vi "LIA_FPGA.vi"() -> ()   [LabVIEW 2010]
uses:
  <vilib>/rvi/LocalResourceManager/LocalResourceManager.xnode
  <vilib>/rvi/DataTransferAndStorage/Container/Common/niFpgaContainerState.ctl
  <vilib>/rvi/DataTransferAndStorage/Container/Common/niFpgaDataTypeControl.ctl
  <vilib>/rvi/DataTransferAndStorage/Container/Common/niFpgaContainerImplementationControl.ctl
  <vilib>/rvi/DataTransferAndStorage/Container/Common/niFpgaContainerArbitrationOptionsControl.ctl
  <vilib>/rvi/DataTransferAndStorage/Container/Common/niFpgaTransferTypeControl.ctl
  <vilib>/rvi/DataTransferAndStorage/Container/Common/niFpgaContainerInitializationParameters.ctl
  <vilib>/rvi/Memory/Memory_Types/niFpgaMemoryInterfaceConfiguration.ctl
  <vilib>/rvi/FIFO/Fifo_Types/niFpgaFifoControlLogicControl.ctl
  <vilib>/rvi/DataTransferAndStorage/Container/Common/niFpgaContainerMetaDataKey.ctl
  <vilib>/Platform/TimedLoop/XDataNode/XDataNode.xnode
  <vilib>/Platform/TimedLoop/XDataNode/timing_clust.ctl
  <vilib>/Platform/TimedLoop/XDataNode/nitl_modes.ctl
  <vilib>/Platform/TimedLoop/XDataNode/wakeup.ctl
  <vilib>/rvi/DataTransferAndStorage/Container/XNode/niFpgaContainer.xnode
  <vilib>/rvi/FXPMathLib/FxpInterpret/XNode/nifxpmath_Interpret.xnode
  <vilib>/eio/EIONode/EIONode.xnode
  <vilib>/rvi/eio/nirviEIOImplementation/nirviEIOImplementation.xnode
  <vilib>/rvi/eio/common/nirviEmuClasses.ctl
  <vilib>/rvi/DataTransferAndStorage/Container/Common/niFpgaContainerGetUniqueNameForEmu.vi
  <vilib>/rvi/DataTransferAndStorage/Container/Common/niFpgaContainerSetEmuInfo.vi
  <vilib>/rvi/eio/common/nirviEmuReportErrorAndStop.vi
  <vilib>/rvi/FIFO/Fifo_Resource/nirvififoEmulationSetSize.vi
  <vilib>/rvi/eio/common/nirviEmuTemplateMethod_noerrors.vi
  <vilib>/Platform/TimedLoop/XDataNode/XDNodeRunTimeDep.lvlib
panel:
  in  "Period":u16=1000
  out "ticks":u16
  out "ref":i16 format="%.0x"
  out "sig":i16 format="%.0x"
  out "channelQ":i64
  out "channelI":i64
  out "f":fxp<+/-,32,0> format="%.32g"
  in  "start":bool
  in  "dec2":i16=1
  in  "K":fxp<+,16,0>=0.001007080078125
  in  "nominal freq":fxp<+,16,0>=0.010009765625
  in  "dec1":i16=1
  in  "stages":i8=1
  in  "stop":bool
  in  "decimation":i16=1024
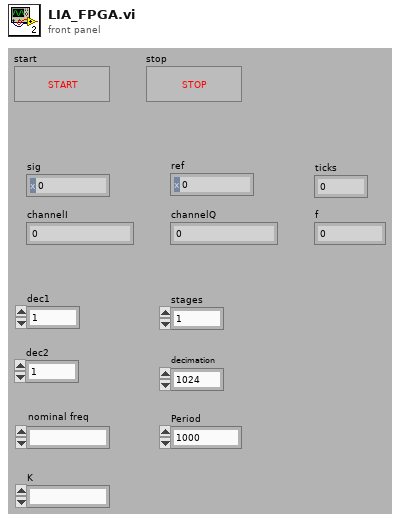
[diagram p1: front panel]
types:
  T1 = typedef "nirviEmuClasses.ctl" = enum16{"IO Read", "IO Write", "Method", "Property Read", "Property Write"}
  T2 = typedef "XDNodeRunTimeDep.lvlib/timing_clust.ctl" = cluster{"Expected End [f-1]":u64, "Actual End [f-1]":u64, "Finished Late? [f-1]":bool, "Expected End [i-1]":u64, "Actual End [i-1]":u64, "Finished Late? [i-1]":bool, "Expected Start [i]":u64, "Actual Start [i]":u64, "Expected Start [f]":u64, "Actual Start [f]":u64, "Source Name":string, "Structure Name":string, "Period":i64, "Deadline":i64, "Offset":i64, "Start":i64, "Priority":i32, "Timeout":i32, "Mode":T3, "Wakeup Reason":T4, "Error":errorcluster, "Source Type":string, "Secondary Source Type":string, "Global End Time":u64, "Global Start Time":u64, "Frame Duration":u64, "Iteration Duration":u64, "Assigned CPU":i32, "I/O Scan Engine Mode":u32}
  T3 = typedef "XDNodeRunTimeDep.lvlib/nitl_modes.ctl" = enum32{"No Change", "Process missed periods, maintain original phase", "Discard missed periods, maintain original phase", "Process missed periods, ignore original phase", "Discard missed periods, ignore original phase"}
  T4 = typedef "XDNodeRunTimeDep.lvlib/wakeup.ctl" = enum32{"Normal", "Aborted", "Asynchronous wakeup", "Timing source error", "Timed loop error", "Timeout"}
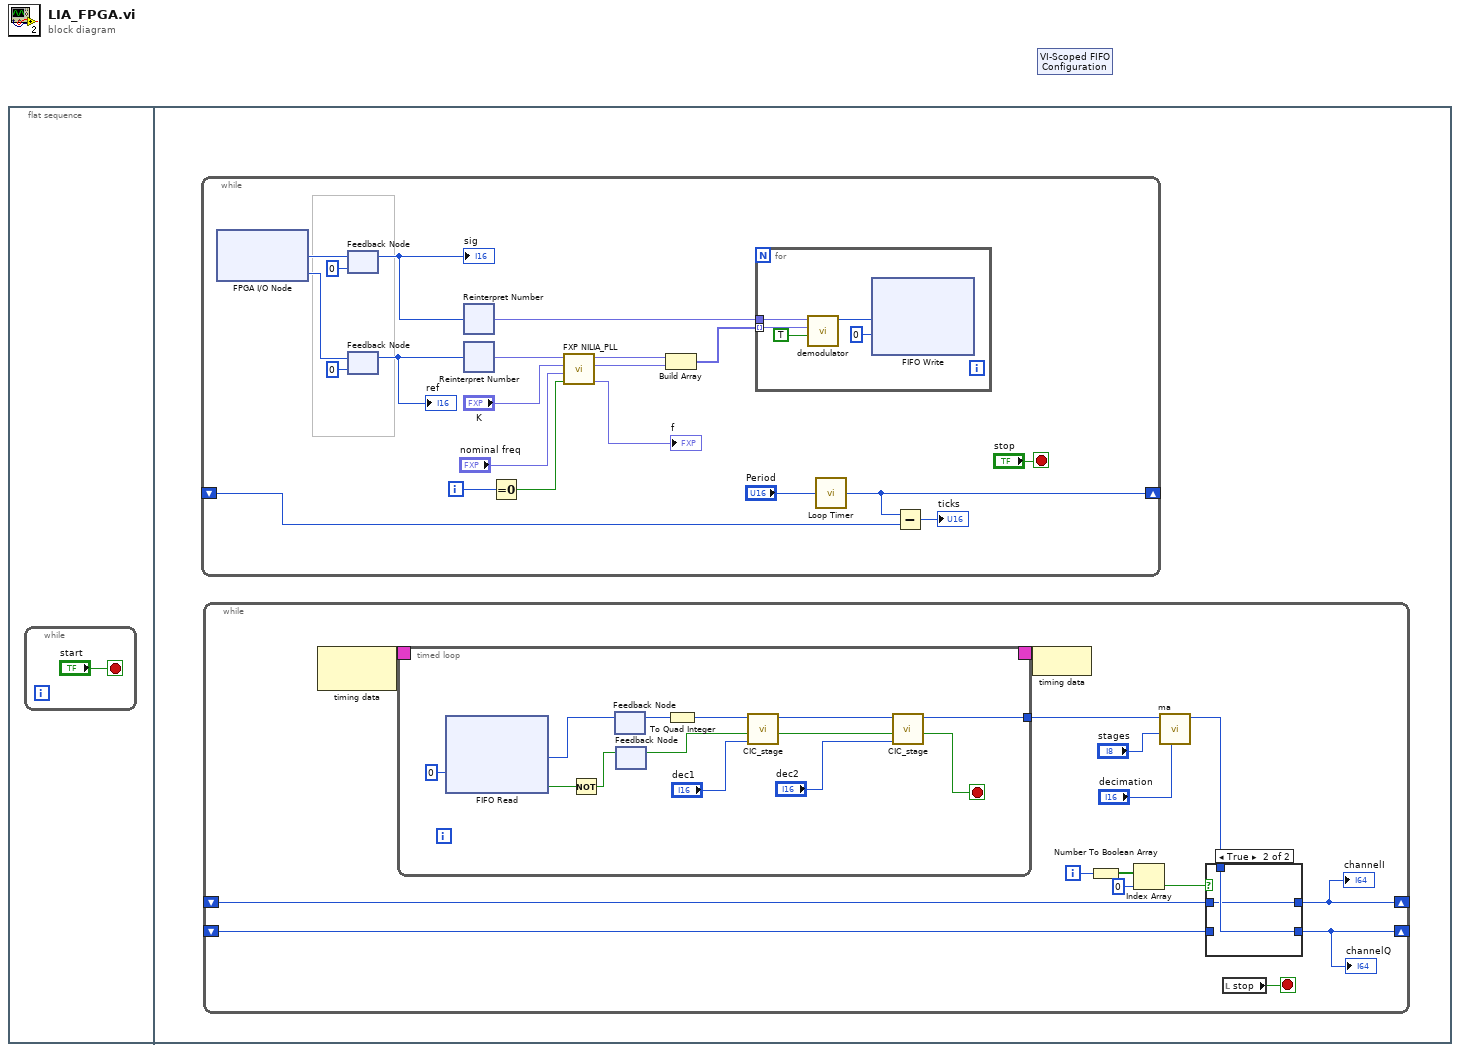
[diagram p0: block diagram]
diagram:
  n1 = flat-sequence {
    frame #0 {
      n2 = while {
        stop <- "start" stop-if-true
      }
    }
    frame #1 {
      n3 = while {
        shift-right: [w15] -> _
        shift-left: _ -> [w14]
        i -> [w22]
        stop <- "stop" stop-if-true
        n4 = xnode "FPGA I/O Node"() -> ("ModA/AI0"=w7:i16, "ModA/AI1"=w4:i16)  [unwired: 2 in, 2 out]
        n5 = feedback #1(i16 0 ("y")) -> (w6:i16)
        "sig" <- w6
        n6 = feedback-in #1(w7) -> ()
        n7 = feedback #2(i16 0 ("z [I32.1]")) -> (w5:i16)
        "ref" <- w5
        n8 = feedback-in #2(w4) -> ()
        n9 = xnode "Reinterpret Number"("x"=w6) -> ("y"=w10:fxp<+/-,16,1>)
        n10 = xnode "Reinterpret Number"("x"=w5) -> ("y"=w12:fxp<+/-,16,1>)
        n11 = Equal To 0?(x=w22) -> (x = 0?=w20:bool)
        n12 = call "FXP NILIA_PLL.vi"("reset?"=w20, "norminal freq [U16.0]"="nominal freq", "alpha [U16.0]"="K", "x[I16.1]"=w12) -> ("f"=→"f":fxp<+/-,32,0>, "sin(z)"=w2:fxp<+/-,16,2>, "cos(z)"=w3:fxp<+/-,16,2>)  [unwired: 1 in, 4 out]
        n13 = Build Array(w3, w2) -> (w11:fxp<+/-,16,2>[])
        n14 = for {
          tunnel: w10 -> [w25]
          tunnel: w11 -> [w23] mode=indexing
          n15 = call "demodulator.vi"("New Data"=TRUE, "ref"=w23, "signal"=w25) -> ("x*y"=w26:i32)  [unwired: 8 out]
          n16 = xnode ("FIFO Write")("Element"=w26, "Timeout"=0) -> ()  [unwired: 1 in, 2 out]
        }
        n17 = call "Loop Timer"("Count(Ticks)"="Period") -> ("Tick Count(Ticks)"=w15:u16)
        n18 = Subtract(x=w15, y=w14) -> (x-y=→"ticks":u16)
      }
      n19 = while {
        shift-right: [w122] -> _
        shift-left: _ -> [w124]
        shift-right: [w121] -> _
        shift-left: _ -> [w123]
        i -> [w129]
        stop <- w131 stop-if-true
        n20 = node-c288() -> (w135:T2)  [unwired: 1 out]
        n21 = timed-loop {
          timing: w135 -> [_]
          timing-out: [_] -> w134
          tunnel: [w143] -> w130
          stop <- w142 stop-if-true
          n22 = xnode ("FIFO Read")("Timeout"=0) -> ("Element"=w150:i32, "Timed Out?"=w149:bool)  [unwired: 1 in, 1 out]
          n23 = Not(x=w149) -> (.not. x?=w148:bool)
          n24 = feedback-in #3(w150) -> ()
          n25 = feedback #3() -> (w152:i32)  [unwired: 1 out]
          n26 = feedback-in #4(w148) -> ()
          n27 = feedback #4() -> (w146:bool)  [unwired: 1 out]
          n28 = To Quad Integer(1:w152) -> (0:w147:i64)
          n29 = call "CIC_stage.vi"("decimate factor"="dec1", "New Data"=w146, "input"=w147) -> ("Data Ready"=w144:bool, "output"=w145:i64)  [unwired: 7 out]
          n30 = call "CIC_stage.vi"("decimate factor"="dec2", "New Data"=w144, "input"=w145) -> ("Data Ready"=w142:bool, "output"=w143:i64)  [unwired: 7 out]
        }
        n31 = node-c288(w134) -> ()
        n32 = Number To Boolean Array(number=w129) -> (Boolean array=w128:bool[])
        n33 = Index Array(array=w128, index=0) -> (element=w126:bool)
        n34 = call "ma.vi"("decimate"="decimation", "stages"="stages", "input"=w130) -> ("output"=w125:i64)  [unwired: 8 out]
        n35 = case shown="True" w126 {
          tunnel: w125 -> [w137 w139]
          tunnel: [w137 w138] -> w122
          tunnel: [w136 w139] -> w121
          tunnel: w124 -> [_ w138]
          tunnel: w123 -> [w136 _]
          frame False {
          }
          frame True {
          }
        }
        "channelI" <- w122
        "channelQ" <- w121
        n36 = local read "stop"() -> (w131:bool)
      }
    }
  }
  n37 = xnode "VI-Scoped FIFO Configuration"() -> ()  [unwired: 1 out]
